vi "Float32Array Destroy.vi"(8 "error in (no error)":errorcluster, 11 "Float32Array DVR in":refnum<data-value>) -> (0 "error out":errorcluster)   [LabVIEW 2015, in "MDSplus.lvlib"]
uses:
  <vilib>/MDSplus/Library/MDSplus.lvlib
  <vilib>/MDSplus/Classes/Data_Class/Array_Class/Float32Array_Class/Float32Array.lvclass
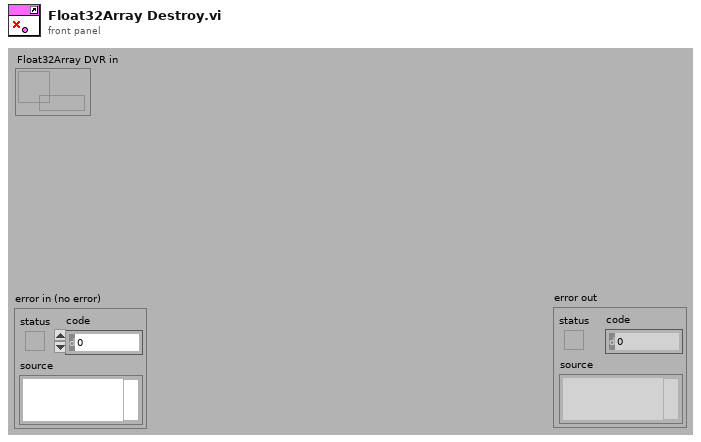
[diagram p1: front panel]
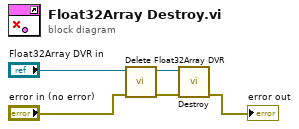
[diagram p0: block diagram]
diagram:
  n1 = call <vilib>:"Delete Float32Array DVR.vi"("error in (no error)"="error in (no error)", "Float32Array DVR in"="Float32Array DVR in") -> ("error out"=w2:errorcluster, "Float32Array out"=w3:refnum<class "Float32Array.lvclass">)  [unwired: 8 in]
  n2 = call-dynamic "Destroy.vi"("error in (no error)"=w2, "Float32Array in"=w3) -> ("error out"=→"error out":errorcluster)  [unwired: 9 in]
